vi "Initialize.vi"(8 "error in (no error)":errorcluster, 11 "Instrument in":refnum<class "Instrument Driver.lvclass">) -> (0 "error out":errorcluster, 3 "Instrument out":refnum<class "Instrument Driver.lvclass">)   [LabVIEW 2020, in "Instrument Driver.lvlib" / "Instrument Driver.lvclass"]
doc: "Initialize the Instrument and set the base configuration."
uses:
  Instrument Driver.lvclass
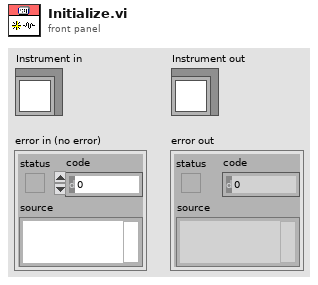
[diagram p1: front panel]
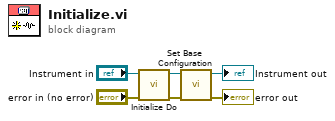
[diagram p0: block diagram]
diagram:
  n1 = call-dynamic "Initialize Do.vi"("error in (no error)"="error in (no error)", "Instrument in"="Instrument in") -> ("error out"=w4:errorcluster, "Instrument out"=w5:refnum<class "Instrument Driver.lvclass">)  [unwired: 8 in]
  n2 = call-dynamic "Set Base Configuration.vi"("error in (no error)"=w4, "Instrument Driver in"=w5) -> ("error out"=→"error out":errorcluster, "Instrument Driver out"=→"Instrument out":refnum<class "Instrument Driver.lvclass">)  [unwired: 8 in]
